vi "Search For Home.vi"(4 "Home mode":T1(ring), 5 "error in (no error)":errorcluster, 7 "Axis (1)":i32=1 min=0 max=3, 8 "VISA resource name":refnum<visa-resource-name>) -> (0 "error out":errorcluster, 3 "VISA resource name out":refnum<visa-resource-name>)   [LabVIEW 2012, in "Newport ESP301.lvlib"]
doc: "This command executes a Home search routine on the axis specified by <B>Axis (1)</B>. If <B>Axis (1)</B>= 0, a home search routine is initiated sequentially on all installed axes. If <B>use current search mode</B> is True, the axes will search for home using the mode specified using <B>set home search mode</B> command.\nIf <B>Home mode</B> = 0, the axes will search for zero position count. If <B>Home mode</B> = 1, the axis will search for combined Home and Index signal transitions. If <B>Home mode</B> = 2, the axes will search for Home signal transition only. If <B>Home mode</B> = 3, the axes will search for positive limit signal transition. If <B>Home mode</B> = 4, the axes will search for negative limit signal transition. If <B>Home mode</B> = 5, the axes will search for positive limit and index signal transition. If <B>Home mode</B> = 6, the axes will search for negative limit and index signal transition.\nAt the end of a home search routine, the position of axes is reset to the value specified using <B>set home preset position</B> command.\nThe home search motion status can be monitored with the Motion Done (MD) status command. If a fault condition such as E-stop occurs while home search is in progress or if this command is issued to an axis before enabling it, the controller returns error xx20, “HOMING ABORTED”.\nFor a detailed description of the home search routine see the Home - The Axis Origin chapter in the Motion Control Tutorial section (ESP301 User's manual.pdf).\n<B>NOTE:</B> This command should be executed once every time the controller power is turned ON or the controller performs a complete system reset. There is no need to issue this command in any other case since the controller always keeps track of position, even when the motor power is OFF.\n<B>NOTE:</B> This command cannot be issued after enabling DAQ (refer ASCII command, DE)."
uses:
  Newport ESP301.lvlib
panel:
  in  "use current search mode (F)":bool
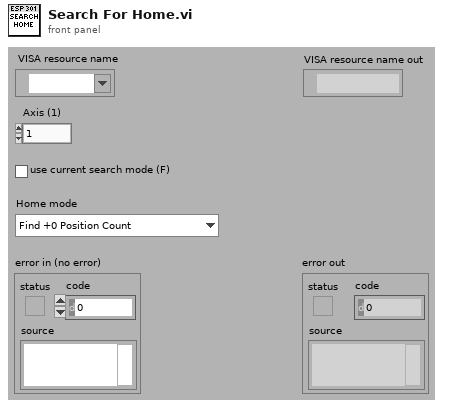
[diagram p1: front panel]
types:
  T1 = enum16{"Find +0 Position Count", "Find Home and Index Signals", "Find Home Signal", "Find Positive Limit Signal", "Find Negative Limit Signal", "Find Positve Limit and Index Signals", "Find Negative Limit and Index Signals"}
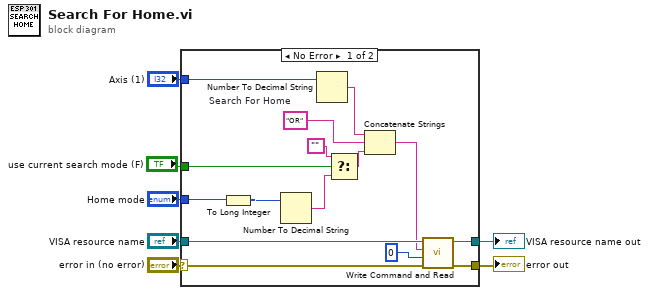
[diagram p0: block diagram]
diagram:
  n1 = case shown="No Error" "error in (no error)" {
    selector: "error in (no error)" -> [w21 w24]
    tunnel: [w20 w24] -> w6
    tunnel: "VISA resource name" -> [w22 w23]
    tunnel: [w19 w23] -> w4
    tunnel: "Axis (1)" -> [w16 _]
    tunnel: "Home mode" -> [w13 _]
    tunnel: "use current search mode (F)" -> [w11 _]
    frame No Error {
      w18 = "OR"  # Search For Home
      n2 = To Long Integer(number=w13) -> (32bit integer=w12:i32)
      n3 = Number To Decimal String(number=w12) -> (decimal integer string=w10:string)  [unwired: 1 in]
      n4 = Number To Decimal String(number=w16) -> (decimal integer string=w17:string)  [unwired: 1 in]
      n5 = Select(t="", s=w11, f=w10) -> (s? t:f=w9:string)
      n6 = Concatenate Strings(w17, w18, w9) -> (w15:string)
      n7 = call "Write Command and Read.vi"("error in (no error)"=w21, "Bytes to read (100)"=u32 0, "Command"=w15, "VISA resource name"=w22) -> ("error out"=w20:errorcluster, "VISA resource name out"=w19:refnum<visa-resource-name>)  [unwired: 3 in, 1 out]
    }
    frame Error {
    }
  }
  "error out" <- w6
  "VISA resource name out" <- w4
